vi "Event Log.Clear Errors.vi"(8 "error in":errorcluster) -> (0 "error out":errorcluster)   [LabVIEW 2024, in "EQMF.lvlib" / "Event Log.lvlib"]
uses:
  Event Log.lvlib
  Queues/Queue Utils.lvlib
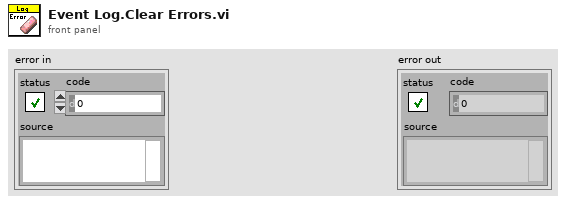
[diagram p1: front panel]
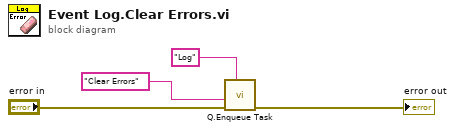
[diagram p0: block diagram]
diagram:
  n1 = call "Q.Enqueue Task.vi"("Q Name"="Log" ("name (unnamed)"), "Error In"="error in", "Task Name"="Clear Errors") -> ("error out"=→"error out":errorcluster)  [unwired: 7 in, 1 out]
